vi "AlliGator Draw Color Map Vertices.vi"(7 "Image Control Refnum":T1 caption="Phasor Plot Display Refnum", 8 "error in (no error)":errorcluster, 9 "Overlay Group":string="Phasor Color Map Contour", 11 "Phasor Plot Refnum in":T2) -> (0 "error out":errorcluster, 3 "Phasor Plot Refnum out":T2)   [LabVIEW 2021, in "AlliGator Phasor Plot Color Map.lvlib"]
doc: "Displays color map vertices on the Phasor Plot."
uses:
  AlliGator Phasor Plot Color Map.lvlib
  <vilib>/vision/Image Controls.llb/IMAQ Image.ctl
  Image/Image Control Refnum.ctl
  Settings/AlliGator Settings List.ctl
  Phasor Ratio/AlliGator Phasor Plot Reference Points.ctl
  Globals, Variables, Constants/AlliGator Variables List.ctl
  Variant/Variant to Data/Variant to Boolean.vi
  Variant/Variant to Data/Variant to I32.vi
  Globals, Variables, Constants/AlliGator Globals, Variables & Constants.lvlib
  Phasor Ratio/AlliGator Phasor Ratio.lvlib
  Settings/AlliGator Settings.lvlib
  Phasor Plot/AlliGator Phasor Plot.lvlib
  Variant/Variant to Data/Variant to Data.lvlib
  Image/Image.lvlib
panel:
  # "see the AlliGator License on the block diagram (Ctrl+E or Window:Show Block Diagram)"
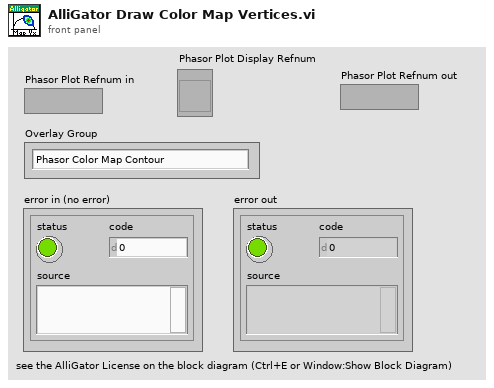
[diagram p1: front panel]
types:
  T1 = typedef "Image.lvlib/Image Control Refnum.ctl" = refnum<vi>
  T2 = typedef "IMAQ Image.ctl" = refnum<image>
  T3 = typedef "AlliGator Settings.lvlib/AlliGator Settings List.ctl" = enum16{"GUI:Visible Settings Tab", "GUI:Last Run Version", "Source Image:Use Image Histogram for Contrast", "Source Image:Low Count Pixels Rejection Options", "Source Image:High Count Pixels Rejection Options", "Source Image:Use Image Brightness", "Source Image:Blend Overlay with Image Background", "Source Image:Use Fixed ROI Diameter", "Source Image:ROI Diameter", "Source Image:ROI Center Color", "Source Image:Peak Threshold", "Source Image:Intensity Threshold", "Source Image:Image Binning Options", "Source Image:Image Smoothing Options", "Source Image:Image Histogram Active", "Source Image:Invert Binary Mask", "Source Image:Hot Pixel Removal", "Source Image:Overlay Analyzed ROI Center", "Source Image:Auto-Adjust Contrast", "Source Image:Histogram Lower Percentile", "Source Image:Histogram Upper Percentile", "Source Image:Save Source Image", "Source Image:Scale Bar Options", "Source Image:Image Resolution (Pixel Size)", "Source Image:Flatfield Correction", "Source Image:Show Dead Left Columns Correction", "Source Image:Dead Left Columns Correction", "Source Image:Image Pre-Processing Operations Order", "Source Image:Overlay ROI Median", "Source Image:Median Overlay Color", "Data Information:Gate Width", "Data Information:Nanotime Gate Separation", "Data Information:Macrotime Gate Separation", "Data Information:Gate Step", "Data Information:# Gates", "Data Information:Gate Image Exposure", "Data Information:Gate Image Integration", "Data Information:Gates to Skip", "Data Information:Gates to Keep", "Data Information:Define Gates to", "Data Information:Channel Name", "Data Information:Available Channel Names", "Data Information:Channel Arithmetic", "Data Information:Background File Subtraction", "Data Information:Background File", "Data Information:Background Scaling Factor", "Data Information:Background Pile-up Correction", "Data Information:Background Pixel Well Capacity", "Data Information:Laser Period", "Data Information:SYNC Period", "Data Information:Pile-up Correction", "Data Information:Pixel Well Capacity", "Data Information:Dataset Scaling Factor", "Fluorescence Decay_Decay Pre-Processing:Reverse Gates", "Fluorescence Decay_Decay Pre-Processing:Verbose Decay Pre-Processing", "Fluorescence Decay_Decay Pre-Processing:Use Decay Pre-Processing", "Fluorescence Decay_Decay Pre-Processing:Background Subtraction", "Fluorescence Decay_Decay Pre-Processing:Background Definition Range", "Fluorescence Decay_Decay Pre-Processing:Baseline Subtraction Method", "Fluorescence Decay_Decay Pre-Processing:Decay Pre-Processing Operations Order", "Fluorescence Decay_Decay Pre-Processing:Smoothing Parameter", "Fluorescence Decay_Decay Pre-Processing:Shift Decay", "Fluorescence Decay_Decay Pre-Processing:Decay Shift Parameters", "Fluorescence Decay_Decay Pre-Processing:Fold Decay", "Fluorescence Decay_Decay Pre-Processing:# Folds", "Fluorescence Decay_Decay Pre-Processing:1-Normalize Decay", "Fluorescence Decay_Decay Pre-Processing:[0-1]-Normalize Decay", "Fluorescence Decay_Decay Pre-Processing:Smoothen Decay", "Fluorescence Decay_Decay Pre-Processing:Extrapolate Decay", "Fluorescence Decay_Decay Pre-Processing:Use Periodicity", "Fluorescence Decay_Decay Pre-Processing:Use Cursors", "Fluorescence Decay_Decay Pre-Processing:Tail Fraction", "Fluorescence Decay_Decay Pre-Processing:Head Fraction", "Fluorescence Decay_Decay Pre-Processing:Additional Points", "Fluorescence Decay_Decay Pre-Processing:Straighten Decay", "Fluorescence Decay_Decay Pre-Processing:Constant Background", "Fluorescence Decay_Decay Pre-Processing:Pixel-Normalize Decay", "Fluorescence Decay_Advanced Analysis:Extract IRF instead of Decay", "Fluorescence Decay_Advanced Analysis:IRF Extraction Options", "Fluorescence Decay_Advanced Analysis:IRF Optimization Options", "Fluorescence Decay_Advanced Analysis:Square Pulse Options", "Fluorescence Decay_Advanced Analysis:IRF Order", "Fluorescence Decay_Advanced Analysis:IRF Time Constants", "Fluorescence Decay_Advanced Analysis:Wavelet Analysis Options", "Fluorescence Decay_Advanced Analysis:Average Lifetime Options", "Fluorescence Decay_Fit Options:Fit Options", "Fluorescence Decay_Fit Options:Use Legacy Fitting Approach", "Fluorescence Decay_Fit Options:Use Data Information Laser Period", "Fluorescence Decay_Fit Parameters:Displayed Fit Parameters", "Fluorescence Decay_Fit Parameters:Fit Parameter Constraints", "Fluorescence Decay_Fit Parameters:Export Tabulated Results", "Fluorescence Decay_Fit Parameters:MLE Baseline Offset Type", "Fluorescence Decay_Fit Parameters:MLE Baseline Offset", "Fluorescence Decay_Fit Parameters:Guess Parameter Names", "Fluorescence Decay_Fit Parameters:Guess Parameter Values", "Fluorescence Decay_Fit Parameters:Guess Parameters Options", "Fluorescence Decay_Styles:Show Last Decay Only", "Fluorescence Decay_Styles:Decay Graph Color Array", "Fluorescence Decay:Decay Graph Active", "Fluorescence Decay Statistics:Min Peak Value", "Fluorescence Decay Statistics:Reject Low Decay Peak Pixels", "Fluorescence Decay Statistics:Reject High Decay Peak Pixels", "Fluorescence Decay Statistics:Max Peak Value", "Time Traces:Use File Timestamp", "Time Traces:Time Step", "Time Traces:Use Intensity Correction File", "Time Traces:Intensity Correction File", "Phasor Plot:Phasor Plot Smoothing Options", "Phasor Plot:Phasor Plot Size", "Phasor Plot:Phasor Plot Graphics Options", "Phasor Plot:Cumulative Phasor Plot", "Phasor Plot:Use Phasor Brightness", "Phasor Plot:Blend Overlay with Phasor Background", "Phasor Plot:Save Phasor Plot", "Phasor Plot:Show References", "Phasor Plot:Phasor Ratio Decay Range", "Phasor Plot:Exponential Fading", "Phasor Plot:Phasor Ratio Reference Colors", "Phasor Plot:Reference Radius", "Phasor Plot:Show Color Map Vertices", "Phasor Plot:Phasor Plot Active", "Phasor Plot:Phasor Ratio Color Map Type", "Phasor Plot:Phasor Ratio Color Map", "Phasor Plot:Phasor Ratio Display Range", "Phasor Plot:Selected Image ROI(s)", "Phasor Plot:All Image ROIs", "Phasor Plot:Selected Phasor Plot ROI(s)", "Phasor Plot:All Phasor Plot ROIs", "Phasor Plot:Phasor Ratio Color-Coded Quantity", "Phasor Plot:Store Phasor Harmonics", "Phasor Plot:Draw Reference Segment", "Phasor Plot:User-Defined Quantity", "Phasor Plot:Color Scale High Color", "Phasor Plot:Color Scale Low Color", "Phasor Graph:Phasor Frequency", "Phasor Graph:Phasor Ratio Type", "Phasor Graph:Pixel-level Phasor Computation", "Phasor Graph:Save Phasor Graph", "Phasor Graph:Phasor Graph Active", "Phasor Graph:Phasor SDV Options", "Phasor Calibration:Use Backup Calibration if needed", "Phasor Graph:Define Shortest Lifetime as", "Phasor Calibration:Backup Calibration Type", "Phasor Calibration:Calibration Type", "Phasor Calibration:Calibration Lifetime", "Phasor Calibration:Calibration Map Algorithm", "Single-Exponential Phasor Locus (SEPL):Gate Parameters", "Single-Exponential Phasor Locus (SEPL):User-defined Gate", "Single-Exponential Phasor Locus (SEPL):User-defined IRF", "Single-Exponential Phasor Locus (SEPL):Phasor Parameters", "Single-Exponential Phasor Locus (SEPL):Decay & IRF Parameters", "Single-Exponential Phasor Locus (SEPL):Display Parameters", "Lifetime Analysis:Decay Analysis Parameters", "Lifetime Analysis:Lifetime Map Active", "Plugins:Python Settings", "Miscellaneous:Verbose Mode", "Miscellaneous:Beep after Script", "Miscellaneous:Saved Image File Format", "Miscellaneous:Exported Gate Image Settings", "Miscellaneous:Include Loading in Timing", "Miscellaneous:Verbose Settings Mode", "Miscellaneous:Histogram Options", "Miscellaneous:Beep on Error", "Miscellaneous:# Logical Processors Used", "Miscellaneous:ROI Description Max Characters", "Miscellaneous:Verbose Error Mode", "Miscellaneous:Transparent Mask Color"}
  T4 = cluster{"Reference 1":u32, "Reference 2":u32, "Boundary":u32}
  T5 = typedef "AlliGator Phasor Ratio.lvlib/AlliGator Phasor Plot Reference Points.ctl" = cluster{"O_h":dbl, "O_v":dbl, "1_h":dbl, "1_v":dbl}
  T6 = typedef "AlliGator Globals, Variables & Constants.lvlib/AlliGator Variables List.ctl" = enum16{"---- GUI ----", "GUI:Initialization Status", "GUI:State Indicators Refnum", "GUI:Original AlliGator Menu Items", "GUI:Current Action Loop State", "GUI:Script in progress", "GUI:Playback", "GUI:Loop Playback", "GUI:Search ROI Used", "GUI:Search ROI", "Decay Graph Max Legend Size", "Intensity Graph Max Legend Size", "Decay Statistics Graph Max Legend Size", "Phasor Graph Max Legend Size", "Phasor Ratio Graph Max Legend Size", "Lifetime Graph Max Legend Size", "---- Files ----", "Files:Export Dataset Frames as Individual Files", "Files:Show Batch Export Help Balloons", "Files:Frames in Dataset", "Files:ptu File Frame Start Indices", "Files:Current Frame in Dataset", "Files:Current Frame Timestamp", "Files:Dataset Loaded", "Files:Dataset Metadata", "Files:Dataset Channel", "Files:Dataset Data Description", "Files:Background Dataset Metadata", "Files:Background Dataset Channel", "Files:Background Dataset Data Description", "Files:Background File Subtraction", "Files:Background File Path", "Files:Background File Pile-up Correction", "Files:Background File Pixel Well Capacity", "Files:Background File Scaling Factor", "Files:Current Dataset Load Settings", "Files:Dataset Path", "Files:ICCD-specific Information", "Files:Macrotime Gate Separation", "------ Python Plugins ------", "Python Plugins:Information", "Python Plugins:Python Session", "Python Plugins:Valid Python Session?", "---- Source Image ----", "Source Image:ROIs", "Source Image:Current ROI", "Source Image:ROI Event Refnum", "X_Source Image:Display Range", "X_Source Image:Palette Information", "X_Source Image:Type of Displayed Image", "X_Time Gate Slider", "Source Image:Palette List", "Source Image:Scale", "Source Image:ROI Overlay Color", "Source Image:Overlay to Erase", "Source Image:Is Displayed Image Accumulated", "Source Image:White Light Image Modified", "Source Image:Mask Image Modified", "---- Image Profile Window ----", "Image Profile:Window Event Refnum", "Image Profile:IntensityType", "Image Profile:Intensity Average Type", "Image Profile:Intensity-weighted SDV", "Image Profile:Box Profile Type", "Image Profile:Window Open", "Image Profile:Plotted Fit Parameter", "------ Phasor Graph -------", "Phasor Graph:Show Line", "---- Phasor Plot ---", "Phasor Plot:Parameters Changed", "Phasor Plot:FLI Dataset Modified since last Calculation", "Phasor Harmonics Data", "Selected Phasor Harmonics", "Phasor Harmonic Manager Event Refnum", "Phasor Plot:ROIs", "Phasor Plot:Current ROI", "Phasor Plot:ROI Event Refnum", "Phasor Plot:Image Reference Points", "Phasor Plot:Computed", "Phasor Plot:Palette Information", "Phasor Plot:Palette List", "Phasor Plot:Phasor Ratio Palette Information", "Phasor Plot:Phasor Ratio Palette List", "Phasor Plot:Image Scale", "Phasor Plot:Image Overlay to Erase", "Phasor Plot:Image Elements to Update", "Phasor Plot:Current Calculation Parameters", "Phasor Plot:Current Calibration Options", "Phasor Plot:Reset Cumulated Phasor Plot", "Phasor Plot:Reference 1", "Phasor Plot:Lifetime Reference 1", "Phasor Plot:Reference 1 Frequency", "Phasor Plot:Reference 2", "Phasor Plot:Lifetime Reference 2", "Phasor Plot:Reference 2 Frequency", "---- Decay Analysis ----", "Number of Selected Decays to Fit", "LS Fit Results", "LAR Fit Results", "BS Fit Results", "Last Decay Max - Min", "Best Fit Parameters", "Best Fit Parameter Names", "Actual Size X", "Actual Size Y", "Binning X", "Binning Y", "Actual # Gates", "Dataset Number", "Gates to...", "Gates Skipped", "Gates to keep", "Gate Step", "Gate Separation", "Reversed Gates", "Pile-up Correction", "Pixel Well Capacity", "Background Subtracted", "Background Subtraction Method", "Background Definition Range", "Background File (deprecated)", "Number of Dataset Accumulated", "Array of Accumulated Dataset Paths", "Do Averaged Datasets", "Destination File Path", "Process Plot Target", "Use 1/D as Phasor Frequency", "---- Decay Fit Parameter Map -----", "Decay Fit Parameter Map:Palette Information", "Decay Fit Parameter Map:Palette List", "---- Parameter Map ----", "Parameter Map:Palette Information", "Parameter Map:Palette List", "------- Local Decay Window ---------", "Local Decay Graph Window:Event Refnum", "Local Decay Graph Window:Use normalized IRF for convolution", "----- Miscellaneous ----", "Misc:Skippable Dialog Windows Status"}
  T7 = cluster{"Phasor Plot x":dbl, "Phasor Plot y":dbl}
  T8 = cluster{"Phasor Plot x":dbl, "Phasor Plot y":dbl}[]
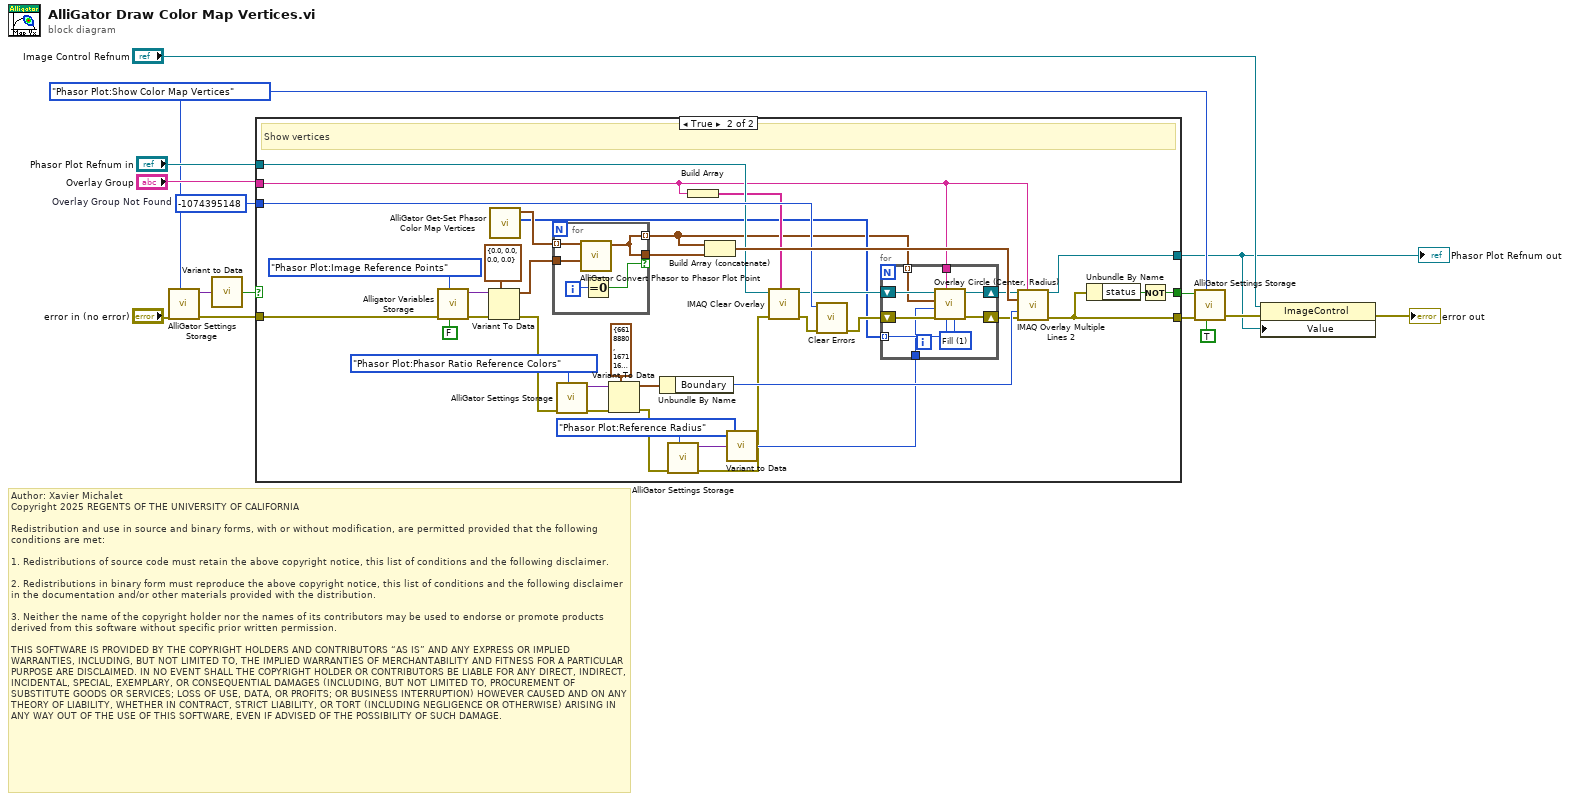
[diagram p0: block diagram]
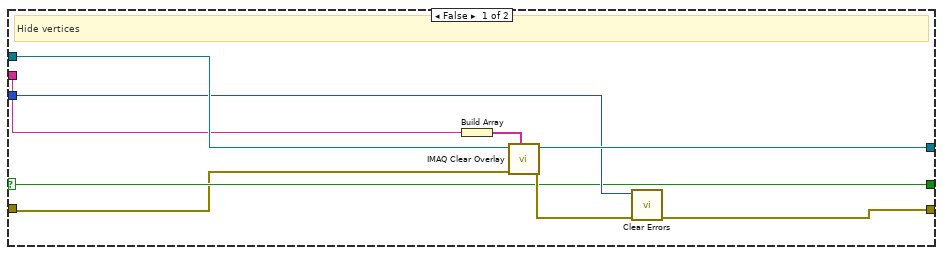
[diagram p2: hidden frame]
diagram:
  w7 = AlliGator_Settings_List."Phasor Plot:Show Color Map Vertices" ("AlliGator Settings List")
  w13 = -1074395148  # Overlay Group Not Found
  # "Author: Xavier Michalet\nCopyright 2025 REGENTS OF THE UNIVERSITY OF CALIFORNIA\n\nRedistribution and use in source and binary forms, with or without modification, are permitted provided that the following conditions are met:\n\n1. Redistributions of source code must retain the above copyright notice, this list of conditions and the following disclaimer.\n\n2. Redistributions in binary form must reproduce the above copyright notice, this list of conditions and the following disclaimer in the documentation and/or other materials provided with the distribution.\n\n3. Neither the name of the copyright holder nor the names of its contributors may be used to endorse or promote products derived from this software without specific prior written permission.\n\nTHIS SOFTWARE IS PROVIDED BY THE COPYRIGHT HOLDERS AND CONTRIBUTORS “AS IS” AND ANY EXPRESS OR IMPLIED WARRANTIES, INCLUDING, BUT NOT LIMITED TO, THE IMPLIED WARRANTIES OF MERCHANTABILITY AND FITNESS FOR A PARTICULAR PURPOSE ARE DISCLAIMED. IN NO EVENT SHALL THE COPYRIGHT HOLDER OR CONTRIBUTORS BE LIABLE FOR ANY DIRECT, INDIRECT, INCIDENTAL, SPECIAL, EXEMPLARY, OR CONSEQUENTIAL DAMAGES (INCLUDING, BUT NOT LIMITED TO, PROCUREMENT OF SUBSTITUTE GOODS OR SERVICES; LOSS OF USE, DATA, OR PROFITS; OR BUSINESS INTERRUPTION) HOWEVER CAUSED AND ON ANY THEORY OF LIABILITY, WHETHER IN CONTRACT, STRICT LIABILITY, OR TORT (INCLUDING NEGLIGENCE OR OTHERWISE) ARISING IN ANY WAY OUT OF THE USE OF THIS SOFTWARE, EVEN IF ADVISED OF THE POSSIBILITY OF SUCH DAMAGE."
  n1 = call "AlliGator Settings Storage.vi"("AlliGator Settings List"=w7, "Error In"="error in (no error)") -> ("Error Out"=w10:errorcluster, "Variant Data out"=w12:variant)  [unwired: 8 in]
  n2 = call-poly "Variant to Data.vi"("Variant"=w12) -> ("Value"=w9:bool)  [unwired: 8 in]
  n3 = case shown="True" w9 {
    selector: w9 -> [w18 _]
    tunnel: w10 -> [w16 w57]
    tunnel: [w17 w40] -> w8
    tunnel: [w24 w45] -> w1
    tunnel: "Overlay Group" -> [w21 w33]
    tunnel: "Phasor Plot Refnum in" -> [w23 w43]
    tunnel: w13 -> [w19 w46]
    tunnel: [w18 w38] -> w6
    frame False {
      # "Hide vertices"
      n4 = Build Array(w21) -> (w22:string[])
      n5 = call "IMAQ Clear Overlay"("Groups"=w22, "error in (no error)"=w16, "Image"=w23) -> ("error out"=w20:errorcluster, "Image Out"=w24:T2)  [unwired: 7 in]
      n6 = call <vilib>:"Clear Errors.vi"("error in (no error)"=w20, "specific error code to clear (0: all)"=w19) -> ("error out"=w17:errorcluster)  [unwired: 4 in, 1 out]
    }
    frame True {
      # "Show vertices"
      n7 = call "Alligator Variables Storage.vi"("Get(F)/Set"=FALSE, "AlliGator Variable"=AlliGator_Variables_List."Phasor Plot:Image Reference Points" ("Alligator Variable"), "Error In"=w57) -> ("Error Out"=w59:errorcluster, "Data out"=w60:variant)  [unwired: 6 in, 1 out]
      n8 = Variant To Data(error in=w59, type=T5 {"O_h"=0.0, "O_v"=0.0, "1_h"=0.0, "1_v"=0.0} ("Phasor Plot Reference Points"), Variant=w60) -> (data=w50:T5, error out=w41:errorcluster)
      n9 = call "AlliGator Get-Set Phasor Color Map Vertices.vi"() -> ("Color Array out"=w31:u32[], "Vertices out"=w32:cluster{"X":dbl, "Y":dbl}[])  [unwired: 8 in, 2 out]
      n10 = for {
        tunnel: w32 -> [w75] mode=indexing
        tunnel: w50 -> [w74]
        tunnel: [w72] -> w25 mode=indexing
        tunnel: [w72] -> w47 if=w71
        i -> [w73]
        n11 = call "AlliGator Convert Phasor to Phasor Plot Point.vi"("Phasor Plot Reference Points"=w74, "Phasor"=w75) -> ("Phasor Plot Point"=w72:T7)  [unwired: 9 in]
        n12 = Equal To 0?(x=w73) -> (x = 0?=w71:bool)
      }
      n13 = call "AlliGator Settings Storage.vi"("AlliGator Settings List"=AlliGator_Settings_List."Phasor Plot:Phasor Ratio Reference Colors", "Error In"=w41) -> ("Error Out"=w52:errorcluster, "Variant Data out"=w54:variant)  [unwired: 8 in]
      n14 = Variant To Data(error in=w52, type=T4 {"Reference 1"=6618880, "Reference 2"=16711680, "Boundary"=16776960} ("Phasor Ratio Reference Colors"), Variant=w54) -> (data=w51:T4, error out=w27:errorcluster)
      n15 = Unbundle By Name(w51) -> ("Boundary"=w48:u32)
      n16 = call "AlliGator Settings Storage.vi"("AlliGator Settings List"=AlliGator_Settings_List."Phasor Plot:Reference Radius", "Error In"=w27) -> ("Error Out"=w26:errorcluster, "Variant Data out"=w29:variant)  [unwired: 8 in]
      n17 = Build Array(w33) -> (w42:string[])
      n18 = Build Array (concatenate)(w25, w47) -> (w49:T8)
      n19 = call-poly "Variant to Data.vi"("Variant"=w29) -> ("Value"=w28:i32)  [unwired: 8 in]
      n20 = call "IMAQ Clear Overlay"("Groups"=w42, "error in (no error)"=w26, "Image"=w43) -> ("error out"=w44:errorcluster, "Image Out"=w35:T2)  [unwired: 7 in]
      n21 = call <vilib>:"Clear Errors.vi"("error in (no error)"=w44, "specific error code to clear (0: all)"=w46) -> ("error out"=w37:errorcluster)  [unwired: 4 in, 1 out]
      n22 = for {
        shift-right: [w69] -> w36
        shift-left: w37 -> [w70]
        shift-right: [w67] -> w34
        shift-left: w35 -> [w68]
        tunnel: w33 -> [w66]
        tunnel: w25 -> [w65] mode=indexing
        tunnel: w31 -> [w64] mode=indexing
        tunnel: w28 -> [w62]
        w63 = u32 1 items=["Frame", "Fill"] ("Drawing Mode (Frame)")
        n23 = call "Overlay Circle (Center, Radius).vi"("Drawing Mode (Frame)"=w63, "Color"=w64, "Overlay Group"=w66, "error in (no error)"=w70, "Radius"=w62, "Center"=w65, "Image Refnum in"=w68) -> ("error out"=w69:errorcluster, "Image Refnum out"=w67:T2)  [unwired: 3 in]
      }
      n24 = call "IMAQ Overlay Multiple Lines 2"("Image"=w34, "Group"=w33, "Line End Points"=w49, "Color"=w48, "error in (no error)"=w36) -> ("Image Out"=w45:T2, "error out"=w40:errorcluster)  [unwired: 9 in]
      n25 = Unbundle By Name(w40) -> ("status"=w39:bool)
      n26 = Not(x=w39) -> (.not. x?=w38:bool)
    }
  }
  "Phasor Plot Refnum out" <- w1
  n27 = call "AlliGator Settings Storage.vi"("Get(F)/Set"=TRUE, "AlliGator Settings List"=w7, "Error In"=w8, "Variant Data in"=w6) -> ("Error Out"=w4:errorcluster)  [unwired: 6 in, 1 out]
  n28 = property class="ImageControl"(reference="Image Control Refnum", error in=w4, "Value"=w1) -> (error out=→"error out":errorcluster)  [unwired: 1 out]
